vi "encodeInt64.vi"(2 "Compress? (T)":bool=TRUE, 3 "Int64":i64) -> (1 "MessagePack":u8[](array[numeric]) format="%.0x")   [LabVIEW 2015, in "MsgPack.lvlib"]
uses:
  MsgPack.lvlib
  encodeInt16.vi
  encodeInt8.vi
  SubVis/encodeFixedInt.vi
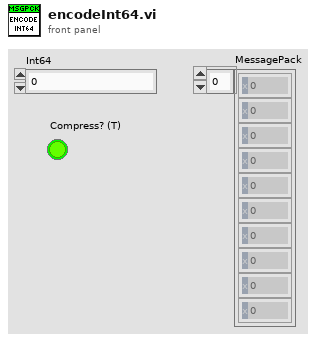
[diagram p1: front panel]
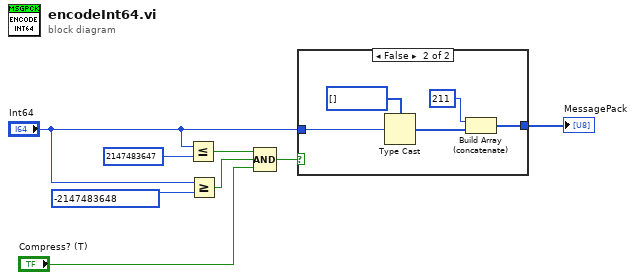
[diagram p0: block diagram]
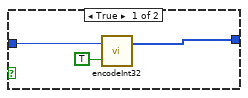
[diagram p2: hidden frame]
diagram:
  n1 = Less Or Equal?(x="Int64", y=i64 2147483647) -> (x <= y?=w6:bool)
  n2 = Greater Or Equal?(x="Int64", y=i64 -2147483648) -> (x >= y?=w5:bool)
  n3 = Compound Arithmetic op=AND(w6, w5, "Compress? (T)") -> (w3:bool)
  n4 = case shown="False" w3 {
    tunnel: [w9 w16] -> w8
    tunnel: "Int64" -> [w10 w12]
    frame True {
      n5 = call "encodeInt32.vi"("Compress? (T)"=TRUE ("Compress"), "Int32"=w10) -> ("MessagePack"=w9:u8[])  [unwired: 1 in]
    }
    frame False {
      n6 = Type Cast(type=u8[] [], x=w12) -> (*(type *) &x=w13:u8[])
      n7 = Build Array (concatenate)(u8 211, w13) -> (w16:u8[])
    }
  }
  "MessagePack" <- w8
